vi "LCSS classification.vi"(9 "cluster centers":string[](array[string])=["1 0 1", "2 0 2", "3 0 3", "4 0 4"], 11 "Patterns in":string[](array[string])=["0 4 0", "4 0 4", "0 4 0", "4 0 4", "0 4 0", "4 0 4", "0 4 0", "4 0 -2", "0 -2 3", "-2 3 0", "3 0 3", "0 3 0", "3 0 4", "0 4 0", "-2 0 1", "0 1 0", "1 0 -4", "0 -4 4", "-2 2 0", "2 0 -1", "0 -1 -4", "-1 -4 1", "-4 1 0", "1 0 3", "0 3 0", "-1 0 -1", "0 -1 2", "0 -1 1", "-1 1 0", "1 0 4", "0 4 0", "4 0 3", "0 3 -2", "3 -2 0", "-2 0 -2", "0 -2 3", "-2 3 -2", "3 -2 0", "-2 0 4", "0 4 0", "4 0 -2", "0 -2 2", "2 -1 0", "-1 0 4", "0 4 0", "4 0 2", "0 2 0", "2 0 -2", "0 -2 0", "1 -1 0", "-1 0 3", "0 3 0", "3 0 -4", "0 -4 4", "-4 4 -4", "4 -4 0", "2 -1 0", "-1 0 3", "0 3 -2", "3 -2 0", "-2 0 -3", "0 -3 0", "-3 0 3", "0 3 0", "3 0 -3", "0 -3 0", "0 4 0", "4 0 4", "0 4 -4", "4 -4 1", "-4 1 -1", "1 -1 0", "-1 0 -3", "0 -3 0", "-3 0 1", "0 1 -4", "1 -4 1", "-4 1 0", "1 0 4", "0 4 0", "4 0 -4", "0 -4 0", "-4 0 -4", "0 -4 4", "-4 4 -4", "4 -4 1", "0 -4 1", "-4 1 0", "1 0 -4", "0 -4 4", "0 4 0", "4 0 -2", "0 -2 2", "-2 2 -2", "2 -2 2", "-2 2 -2", "2 -2 2", "-2 2 -1", "2 -1 0", "-1 0 4", "0 4 0", "4 0 2", "0 2 0", "2 0 4", "0 4 0", "4 0 2", "0 2 -2", "2 -2 0", "-2 0 4", "1 0 -1", "0 -1 0", "-1 0 -1", "0 -1 0", "-1 0 1", "0 1 -1", "-2 2 -2", "2 -2 3", "1 0 -1", "0 -1 0", "-1 0 -1", "0 -1 2", "-1 2 0", "2 0 2", "0 2 -2", "2 -2 0", "-2 0 -4", "0 -4 0", "-2 2 0", "2 0 3", "0 3 -2", "3 -2 2", "1 -1 0", "-1 0 3", "0 4 0", "-2 0 1", "0 1 -4", "1 -4 0", "-4 0 -3", "0 -3 0", "1 0 -1", "0 -1 2", "-1 2 -1", "2 -1 1", "-1 1 -4", "-2 0 -1", "0 -1 1", "0 3 0", "3 0 3", "0 3 0", "3 0 3", "0 3 -2", "-4 0 -4", "0 -4 4", "0 4 0", "4 0 -4", "0 -4 0", "-4 0 -4", "-2 2 0", "2 0 4", "0 4 -4", "4 -4 0", "-4 0 2", "0 2 -2"]) -> (0 "Assigned cluster (0) unassigned":string[](array[string]), 1 "patterns in, distance values":string[][](array[string]), 3 "Cluster element count":i32[](array[numeric]))   [LabVIEW 2013]
panel:
  out "Distance values (LCS)":dbl[][](array[numeric])
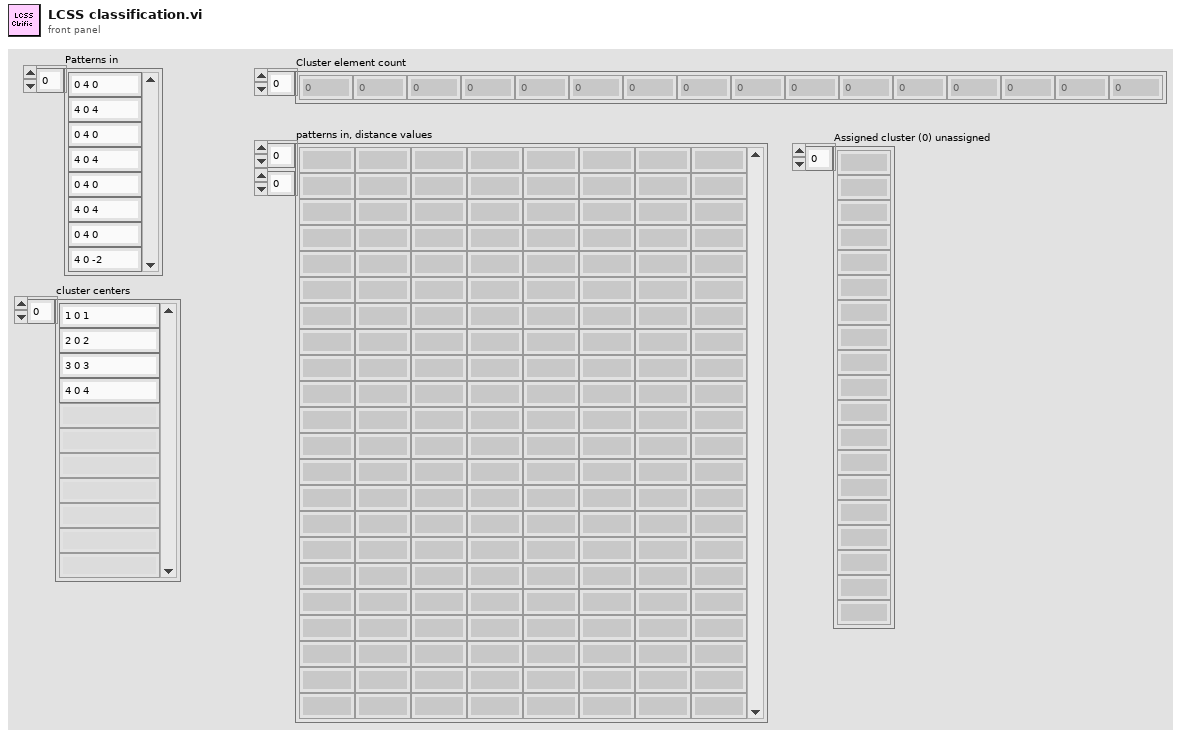
[diagram p1: front panel]
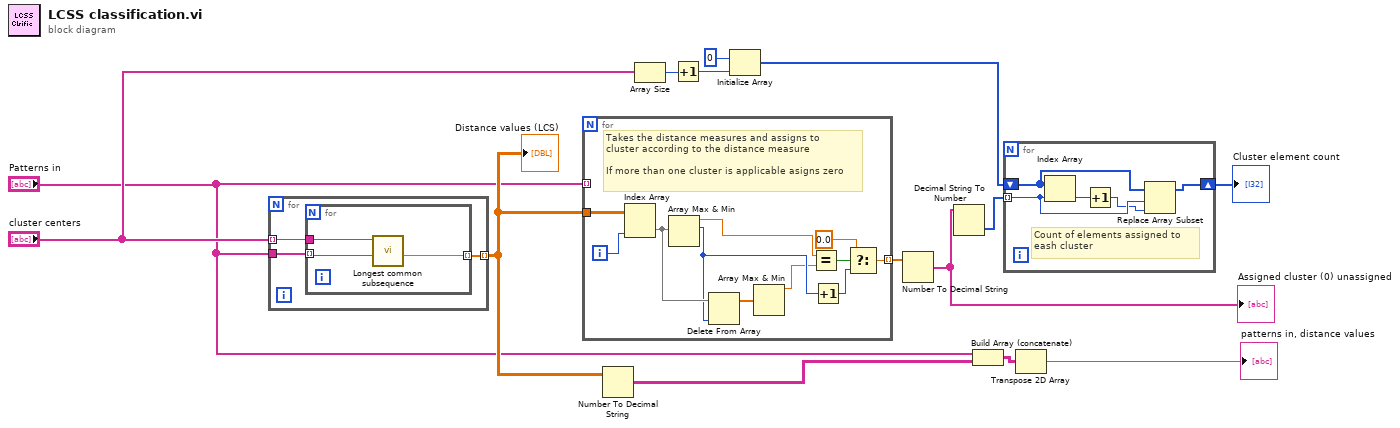
[diagram p0: block diagram]
diagram:
  n1 = for {
    tunnel: "cluster centers" -> [w17] mode=indexing
    tunnel: [w16] -> w9 mode=indexing
    tunnel: "Patterns in" -> [w15]
    n2 = for {
      tunnel: w15 -> [w19] mode=indexing
      tunnel: w17 -> [w20]
      tunnel: [w18] -> w16 mode=indexing
      n3 = call "Longest common subsequence.vi"("Pattern 2 COLUMN(0)"=w19, "Pattern 1 ROW(0)"=w20) -> ("LCS length"=w18:dbl)  [unwired: 8 in, 1 out]
    }
  }
  "Distance values (LCS)" <- w9
  n4 = for {
    tunnel: "Patterns in" -> [_] mode=indexing
    tunnel: w9 -> [w31]
    tunnel: [w21] -> w14 mode=indexing
    i -> [w30]
    # "Takes the distance measures and assigns to \ncluster according to the distance measure\n\nIf more than one cluster is applicable asigns zero"
    n5 = Index Array(array=w31, index (col)=w30) -> (element=w25:dbl[])  [unwired: 1 in]
    n6 = Array Max & Min(array=w25) -> (max value=w24:dbl, max index (indices)=w23:i32)  [unwired: 2 out]
    n7 = Delete From Array(array=w25, index=w23) -> (array with subset deleted=w29:dbl[])  [unwired: 1 in, 1 out]
    n8 = Array Max & Min(array=w29) -> (max value=w22:dbl)  [unwired: 3 out]
    n9 = Equal?(x=w24, y=w22) -> (x = y?=w28:bool)
    n10 = Increment(x=w23) -> (x+1=w26:i32)
    n11 = Select(t=0.0, s=w28, f=w26) -> (s? t:f=w21:dbl)
  }
  n12 = Number To Decimal String(number=w9) -> (decimal integer string=w7:string[][])  [unwired: 1 in]
  n13 = Array Size(array="cluster centers") -> (size(s)=w4:i32)
  n14 = Increment(x=w4) -> (x+1=w3:i32)
  n15 = Initialize Array(0 ("index"), w3) -> (w2:i32[])
  n16 = Number To Decimal String(number=w14) -> (decimal integer string=w8:string[])  [unwired: 1 in]
  "Assigned cluster (0) unassigned" <- w8
  n17 = Decimal String To Number(string=w8) -> (number=w12:i32[])  [unwired: 2 in, 1 out]
  n18 = Build Array (concatenate)("Patterns in", w7) -> (w13:string[][])
  n19 = for {
    tunnel: w12 -> [w34] mode=indexing
    shift-right: [w32] -> w11
    shift-left: w2 -> [w35]
    # "Count of elements assigned to \neash cluster"
    n20 = Index Array(array=w35, index=w34) -> (element=w36:i32)
    n21 = Increment(x=w36) -> (x+1=w33:i32)
    n22 = Replace Array Subset(array=w35, new element=w33, index=w34) -> (w32:i32[])
  }
  "Cluster element count" <- w11
  n23 = Transpose 2D Array(2D array=w13) -> (transposed array=→"patterns in, distance values":string[][])
